vi "Set Refs For UserInfo.vi"(8 "error in (no error)":errorcluster, 10 "Refs":T1, 11 "MemberInfo in":refnum<class "Information.lvclass">) -> (0 "error out":errorcluster, 3 "MemberInfo out":refnum<class "Information.lvclass">)   [LabVIEW 2015, in "Member_Actor.lvlib" / "Information.lvclass"]
uses:
  Information.lvclass
  Type Definitions/Main Ctl and VI ref.ctl
  Information.lvclass/Information.ctl
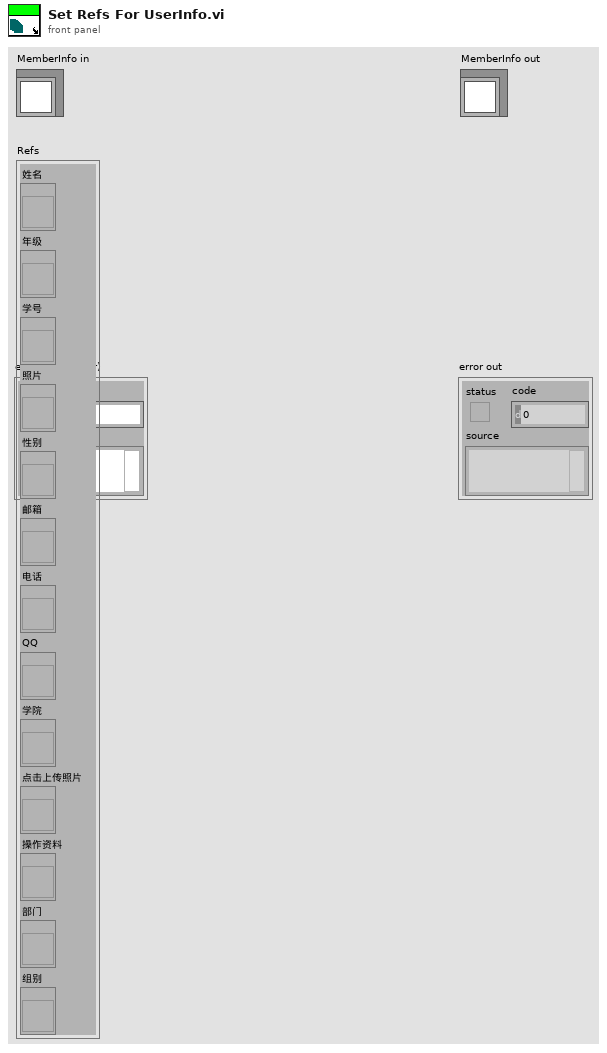
[diagram p1: front panel]
types:
  T1 = typedef "Member_Actor.lvlib/Information.lvclass/Main Ctl and VI ref.ctl" = cluster{"姓名":refnum<vi>, "年级":refnum<vi>, "学号":refnum<vi>, "照片":refnum<vi>, "性别":refnum<vi>, "邮箱":refnum<vi>, "电话":refnum<vi>, "QQ":refnum<vi>, "学院":refnum<vi>, "点击上传照片":refnum<vi>, "操作资料":refnum<vi>, "部门":refnum<vi>, "组别":refnum<vi>}
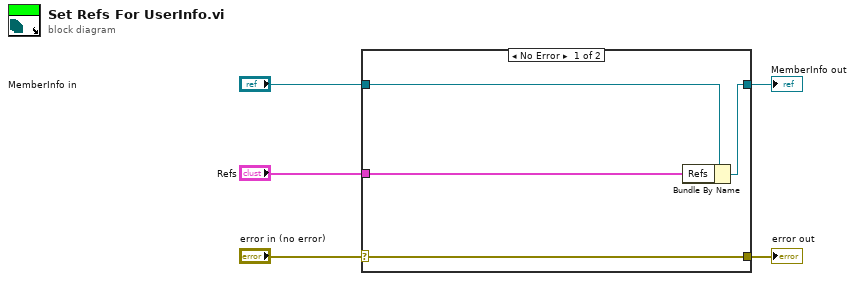
[diagram p0: block diagram]
diagram:
  n1 = case shown="No Error" "error in (no error)" {
    selector: "error in (no error)" -> [w9 w10]
    tunnel: [w9 w10] -> w4
    tunnel: [w7 w11] -> w2
    tunnel: "MemberInfo in" -> [w8 w11]
    tunnel: "Refs" -> [w6 _]
    frame No Error {
      n2 = Bundle By Name(cluster=w8, "Refs"=w6) -> (w7:refnum<class "Information.lvclass">)
    }
    frame Error {
    }
  }
  "error out" <- w4
  "MemberInfo out" <- w2
